vi "getCapacitance.vi"(8 "error in (no error)":errorcluster, 11 "Inst.AH2500 in":refnum<class "Inst.AH2500.lvclass">) -> (0 "error out":errorcluster, 2 "Capacitance (pF)":dbl, 3 "Inst.AH2500 out":refnum<class "Inst.AH2500.lvclass">)   [LabVIEW 2019, in "Inst.AH2500.lvclass"]
uses:
  Inst.AH2500.lvclass
  C:/Program Files (x86)/National Instruments/LabVIEW 2019/user.lib/LevyLab/Instrument Framework/SMOs/Instrument/Instrument.lvclass
  Typedefs/Inst.AH2500.Commands--Enum.ctl
  Typedefs/Inst.AH2500.getAll--Cluster.ctl
  <userlib>/LevyLab/Instrument Framework/SMOs/Instrument/Instrument.lvclass/Instrument.ctl
  991804cd-2d63-4689-a149-8f7b841441b7.vi
  991804cd-2d63-4689-a149-8f7b841441b7.vi/e53b5264-71fb-48ab-b0d1-349ac1055fbe.vi
  991804cd-2d63-4689-a149-8f7b841441b7.vi/e53b5264-71fb-48ab-b0d1-349ac1055fbe.vi/99a3c977-aac1-43c7-9b5c-104fd6873bd3.vi
  <userlib>/LevyLab/Instrument Framework/SMOs/Instrument/API/Send and Receive.vi
  991804cd-2d63-4689-a149-8f7b841441b7.vi/e53b5264-71fb-48ab-b0d1-349ac1055fbe.vi/f1c5cd8d-6986-47d3-bda1-87a5f1c2150e.vi
  <userlib>/LevyLab/Instrument Framework/SMOs/Instrument/Private/Get Client Type.vi
  991804cd-2d63-4689-a149-8f7b841441b7.vi/e53b5264-71fb-48ab-b0d1-349ac1055fbe.vi/99a3c977-aac1-43c7-9b5c-104fd6873bd3.vi/21a019d4-7024-4b1d-a0a8-1ffad19c3b46.vi
  991804cd-2d63-4689-a149-8f7b841441b7.vi/e53b5264-71fb-48ab-b0d1-349ac1055fbe.vi/99a3c977-aac1-43c7-9b5c-104fd6873bd3.vi/a86f4706-720b-4342-95b4-a8fedc6245b7.vi
  991804cd-2d63-4689-a149-8f7b841441b7.vi/e53b5264-71fb-48ab-b0d1-349ac1055fbe.vi/f1c5cd8d-6986-47d3-bda1-87a5f1c2150e.vi/2665ec99-f579-41e3-941f-a2b489b35b67.vi
  991804cd-2d63-4689-a149-8f7b841441b7.vi/e53b5264-71fb-48ab-b0d1-349ac1055fbe.vi/f1c5cd8d-6986-47d3-bda1-87a5f1c2150e.vi/31842105-26dc-4939-bf38-79d624032a51.vi
  991804cd-2d63-4689-a149-8f7b841441b7.vi/e53b5264-71fb-48ab-b0d1-349ac1055fbe.vi/f1c5cd8d-6986-47d3-bda1-87a5f1c2150e.vi/2665ec99-f579-41e3-941f-a2b489b35b67.vi/3254c563-1a36-4944-b86e-9d6365108caa.vi
  991804cd-2d63-4689-a149-8f7b841441b7.vi/e53b5264-71fb-48ab-b0d1-349ac1055fbe.vi/f1c5cd8d-6986-47d3-bda1-87a5f1c2150e.vi/2665ec99-f579-41e3-941f-a2b489b35b67.vi/9d7d0063-afde-4297-8fc3-328c732ff14e.vi
  <userlib>/LevyLab/Instrument Framework/SMOs/Instrument/Private/Get RC Connection Status.vi
  <userlib>/LevyLab/Instrument Framework/SMOs/Instrument/API/Enum to String.vi
  <userlib>/LevyLab/Instrument Framework/SMOs/RemoteControl/API/Send and Receive.vi
  <vilib>/Utility/Data Type/Get Type Information.vi
  <vilib>/JDP Science/JSONtext/JSON text to Variant.vi
  <userlib>/LevyLab/Instrument Framework/SMOs/Instrument/API/Instrument.GetPublicEvents.vi
  <vilib>/JDP Science/JSONtext/Variant to JSON Text.vi
  <vilib>/National Instruments/GUID Generator/Guid Generator.vi
  <userlib>/LevyLab/Instrument Framework/SMOs/Instrument/API/Instrument.MessageToProcess.vi
  <userlib>/LevyLab/Instrument Framework/SMOs/Instrument/Private/Instrument.MessageFromProcess.EventStructure.vi
  <vilib>/JDP Science/JSONtext/LVClass Serializer/JSONtext LVClass Serializer.lvclass
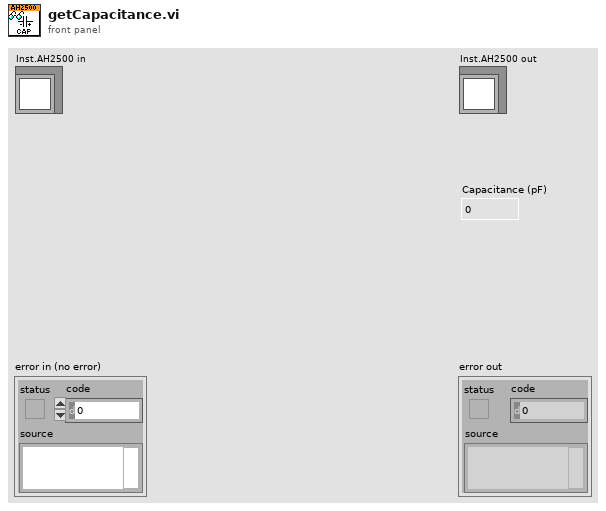
[diagram p1: front panel]
types:
  T1 = typedef "Inst.AH2500.lvclass/Inst.AH2500.getAll--Cluster.ctl" = cluster{"capacitance (pF)":dbl, "loss (nS)":dbl, "Vexc (V)":dbl}
  T2 = typedef "Inst.AH2500.lvclass/Inst.AH2500.Commands--Enum.ctl" = enum16{"getCapacitance", "getLoss", "getExcitation"}
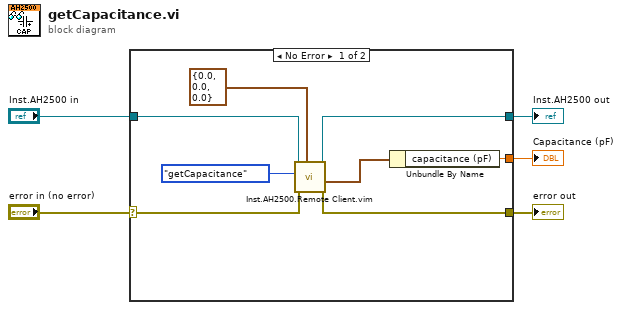
[diagram p0: block diagram]
diagram:
  n1 = case shown="No Error" "error in (no error)" {
    selector: "error in (no error)" -> [w11 w15]
    tunnel: [w10 w15] -> w4
    tunnel: [w8 w14] -> w3
    tunnel: [w13 _] -> w2
    tunnel: "Inst.AH2500 in" -> [w7 w14]
    frame No Error {
      n2 = call "Inst.AH2500.Remote Client.vim"("Data Out type"=T1 {"capacitance (pF)"=0.0, "loss (nS)"=0.0, "Vexc (V)"=0.0} ("getAll"), "error in (no error)"=w11, "Commands"=Inst.AH2500.Commands--Enum."getCapacitance", "Inst.AH2500 in"=w7) -> ("error out"=w10:errorcluster, "Data out"=w9:T1, "Inst.AH2500 out"=w8:refnum<class "Inst.AH2500.lvclass">)  [unwired: 5 in]
      n3 = Unbundle By Name(w9) -> ("capacitance (pF)"=w13:dbl)
    }
    frame Error {
    }
  }
  "error out" <- w4
  "Inst.AH2500 out" <- w3
  "Capacitance (pF)" <- w2
